vi "Set Channel Enable.vi"(8 "error in (no error)":errorcluster, 9 "Channel Enable":bool, 10 "idxChannel":i32, 11 "hdwf":i32) -> (0 "error out":errorcluster)   [LabVIEW 2024, in "AD2 DLL.lvlib"]
uses:
  AD2 DLL.lvlib
  <vilib>/Digilent/AD2 Toolkit/AD2.lvlib
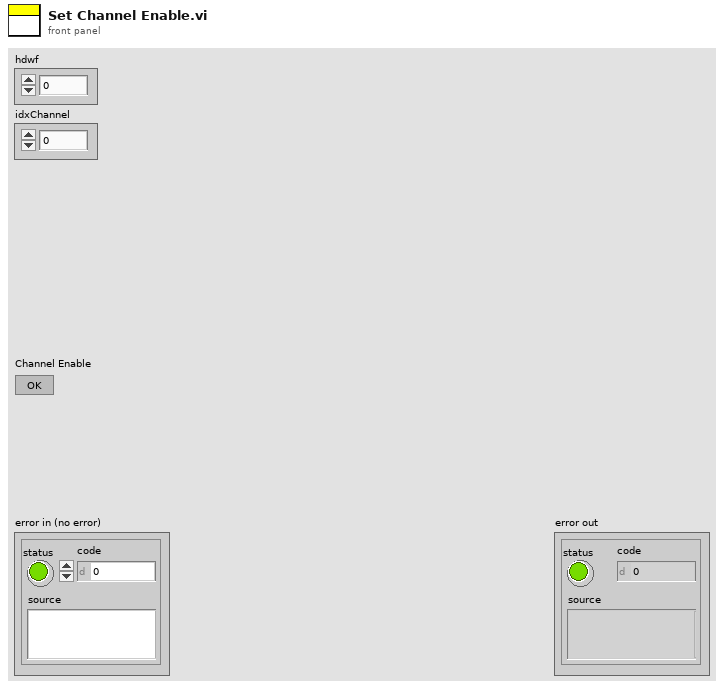
[diagram p1: front panel]
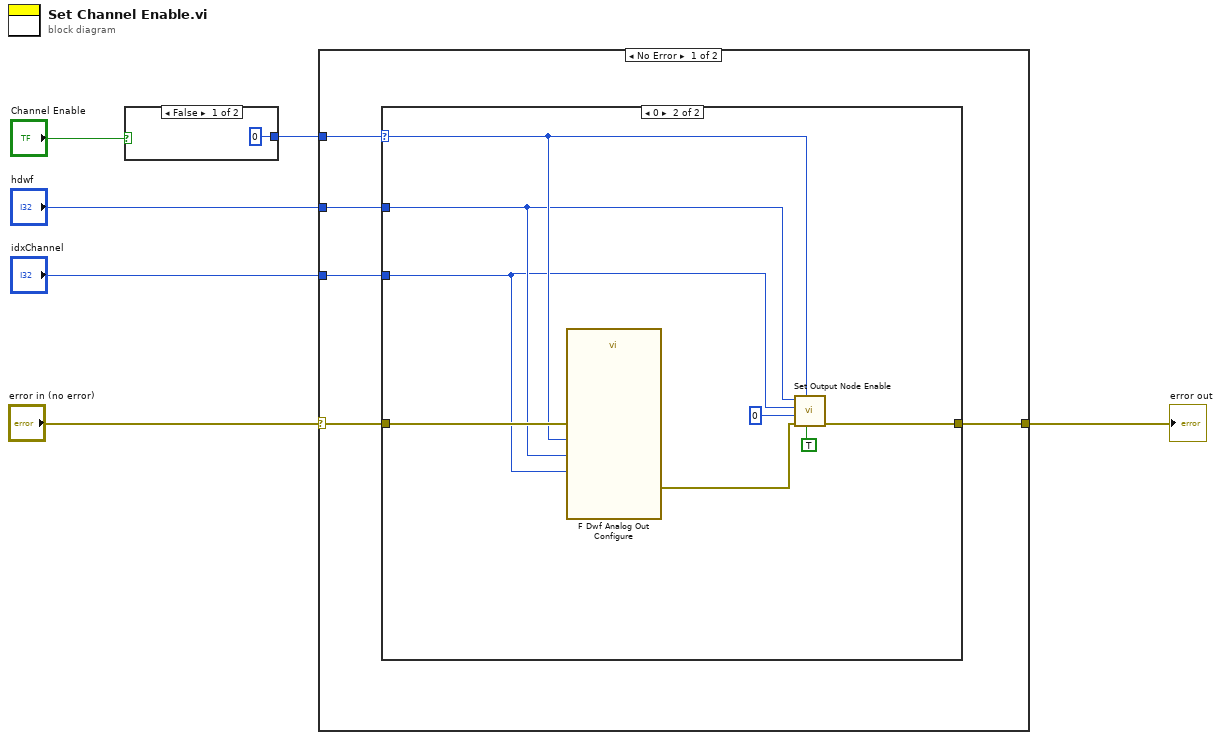
[diagram p0: block diagram]
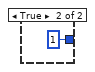
[diagram p2: hidden frame]
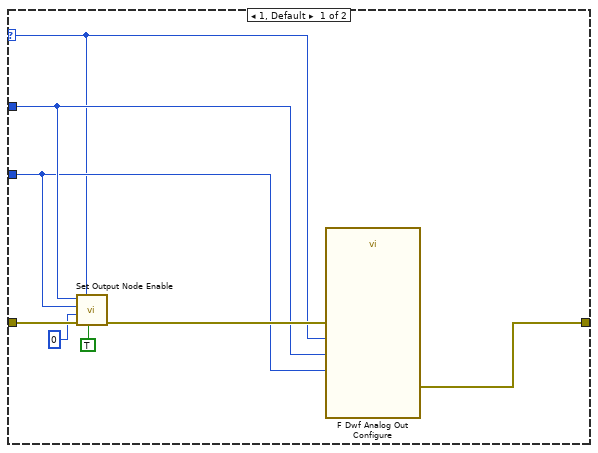
[diagram p3: hidden frame]
diagram:
  n1 = case shown="False" "Channel Enable" {
    tunnel: [0 ("fStart") 1 ("fStart")] -> w3
    frame False {
    }
    frame True {
    }
  }
  n2 = case shown="No Error" "error in (no error)" {
    selector: "error in (no error)" -> [w12 w30]
    tunnel: [w13 w30] -> w6
    tunnel: w3 -> [w9 _]
    tunnel: "hdwf" -> [w11 _]
    tunnel: "idxChannel" -> [w10 _]
    frame No Error {
      n3 = case shown="0" w9 {
        selector: w9 -> [w14 w24]
        tunnel: [w21 w25] -> w13
        tunnel: w12 -> [w20 w27]
        tunnel: w11 -> [w18 w23]
        tunnel: w10 -> [w17 w22]
        frame 1, Default {
          n4 = call "Set Output Node Enable.vi"("Update"=TRUE, "Enable"=w14, "error in (no error)"=w20, "node"=0, "idxChannel"=w17, "hdwf"=w18) -> ("error out"=w19:errorcluster)  [unwired: 4 in, 1 out]
          n5 = call <vilib>:"F Dwf Analog Out Configure.vi"("error in (no error)"=w19, "fStart"=w14, "idxChannel"=w17, "hdwf"=w18) -> ("error out"=w21:errorcluster)  [unwired: 6 in, 1 out]
        }
        frame 0 {
          n6 = call <vilib>:"F Dwf Analog Out Configure.vi"("error in (no error)"=w27, "fStart"=w24, "idxChannel"=w22, "hdwf"=w23) -> ("error out"=w26:errorcluster)  [unwired: 6 in, 1 out]
          n7 = call "Set Output Node Enable.vi"("Update"=TRUE, "Enable"=w24, "error in (no error)"=w26, "node"=0, "idxChannel"=w22, "hdwf"=w23) -> ("error out"=w25:errorcluster)  [unwired: 4 in, 1 out]
        }
      }
    }
    frame Error {
    }
  }
  "error out" <- w6
